vi "Link Control References.vi"(8 "error in":errorcluster, 10 "Control Map":T1[](array[typedef]), 11 "MLTFNC in":refnum<class "MLTFNC.lvclass">) -> (0 "error out":errorcluster, 3 "MLTFNC out":refnum<class "MLTFNC.lvclass">)   [LabVIEW 2019, in "MLTFNC.lvlib" / "MLTFNC.lvclass"]
uses:
  Library/MLTFNC.lvclass
  builds/Instruments/Instruments.lvlibp/Custom Controls/Control Element.ctl
  Library/MLTFNC.lvclass/MLTFNC.ctl
  builds/Instruments/Instruments.lvlibp/Library/Instruments.lvclass
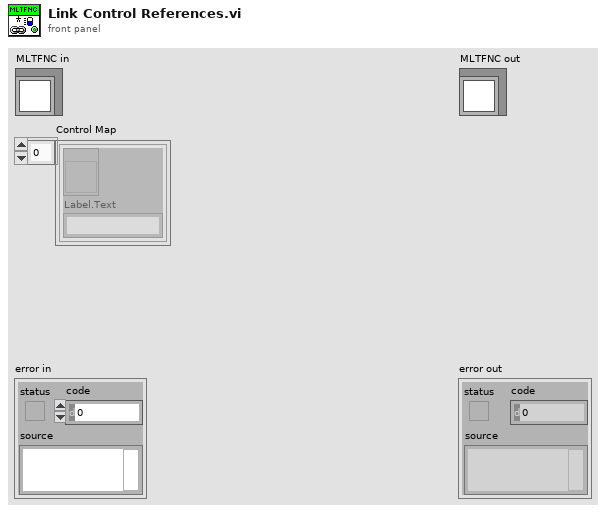
[diagram p1: front panel]
types:
  T1 = typedef "Instruments.lvlibp/Instruments.lvclass/Control Element.ctl" = cluster{refnum<vi>, "Label.Text":string}
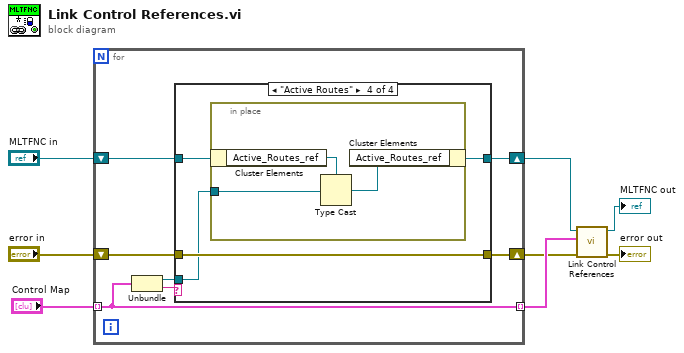
[diagram p0: block diagram]
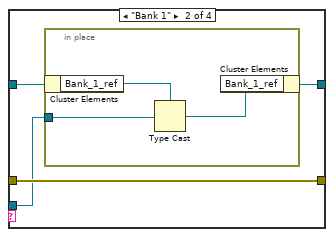
[diagram p3: hidden frame]
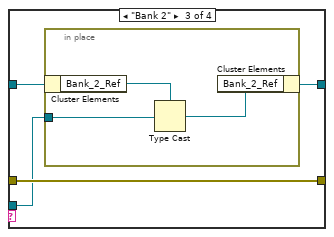
[diagram p4: hidden frame]
diagram:
  n1 = for {
    shift-right: [w9] -> w5
    shift-left: "MLTFNC in" -> [w12]
    tunnel: "Control Map" -> [w13] mode=indexing
    tunnel: [w13] -> w3 mode=indexing
    shift-right: [w10] -> w1
    shift-left: "error in" -> [w11]
    n2 = Unbundle(w13) -> (w14:refnum<vi>, "Label.Text"=w15:string)
    n3 = case shown="\"Active Routes\"" w15 {
      tunnel: w14 -> [_ w18 w25 w32]
      tunnel: w12 -> [w17 w20 w27 w34]
      tunnel: w11 -> [w16 w21 w28 w35]
      tunnel: [w16 w21 w28 w35] -> w10
      tunnel: [w17 w19 w26 w33] -> w9
      frame Default {
      }
      frame "Bank 1" {
        n4 = in-place {
          in-place-border: w18 -> [w24]
          n5 = in-place-cluster #1(w20) -> ("Bank_1_ref"=w23:refnum<vi>)
          n6 = Type Cast(type=w23, x=w24) -> (*(type *) &x=w22:refnum<vi>)
          n7 = in-place-cluster #1("Bank_1_ref"=w22) -> (w19:refnum<class "MLTFNC.lvclass">)
        }
      }
      frame "Bank 2" {
        n8 = in-place {
          in-place-border: w25 -> [w31]
          n9 = in-place-cluster #2(w27) -> ("Bank_2_Ref"=w30:refnum<vi>)
          n10 = Type Cast(type=w30, x=w31) -> (*(type *) &x=w29:refnum<vi>)
          n11 = in-place-cluster #2("Bank_2_Ref"=w29) -> (w26:refnum<class "MLTFNC.lvclass">)
        }
      }
      frame "Active Routes" {
        n12 = in-place {
          in-place-border: w32 -> [w38]
          n13 = in-place-cluster #3(w34) -> ("Active_Routes_ref"=w37:refnum<vi>)
          n14 = Type Cast(type=w37, x=w38) -> (*(type *) &x=w36:refnum<vi>)
          n15 = in-place-cluster #3("Active_Routes_ref"=w36) -> (w33:refnum<class "MLTFNC.lvclass">)
        }
      }
    }
  }
  n16 = call-parent "Link Control References.vi"("error in (no error)"=w1, "Control Map"=w3, "Instruments in"=w5) -> ("error out"=→"error out":errorcluster, "Instruments out"=→"MLTFNC out":refnum<class "MLTFNC.lvclass">)  [unwired: 7 in]
